vi "main_remote.vi"() -> ()   [LabVIEW 2019]
uses:
  Ctrl/status.ctl
  Ctrl/cmd_common.ctl
  Ctrl/udp_item.ctl
panel:
  out "Lat Long":cluster{"Lat":dbl, "Long":dbl} {"Lat" format="%.8f"; "Long" format="%.8f"}
  out "Batt":dbl(slide) scale=25.0..29.0
  out "Velocity feedback":cluster{"VL-p":dbl, "VA-p":dbl} {"VL-p" scale=-1.0..1.0; "VA-p" scale=-1.0..1.0}
  out "Error Display":T2={"AGV"=2, "AGV Estop"=0, "Obstacle"=2, "GNSS"=1, "TIM571"=1, "Cam"=2, "Joystick"=0}
  out "Connection":i32(ring)=1
  in  "close":bool
  in  "Start":bool
  in  "Stop":bool
  in  "tap UI":enum32{"Main", "Config"}(tab)
  out "Joystick":cluster{"X":dbl, "Y":dbl}[](graph)=[{"X"=0.0, "Y"=0.0}, {"X"=-0.0007812738425855281, "Y"=-0.008435316019165624}]
  in  "agv control":T3
  out "Image 3":T4(plugin-control)
  in  "Joystick cfg":T5={"X axis max"=0.0, "X axis min"=0.0, "Y axis max"=0.0, "Y axis min"=0.0, "Speed-out_max"=0.0, "Speed-out_min"=0.0, "Steer-out_max"=0.0, "Steer-out_min"=0.0, "Joystick ID"=0, "joystick scale"=327670}
  in  "udp cfg":T6={"local port"=61556, "remote port"=61550, "RBA IP"="192.168.1.34"}
  out "udp r buff out":string
  in  "RBA status":string
  out "speed_feedback":cluster{"X":dbl, "Y":dbl}[](graph)=[{"X"=0.0, "Y"=0.0}, {"X"=-0.0007812738425855281, "Y"=-0.008435316019165624}]
  # "SRC Remote"
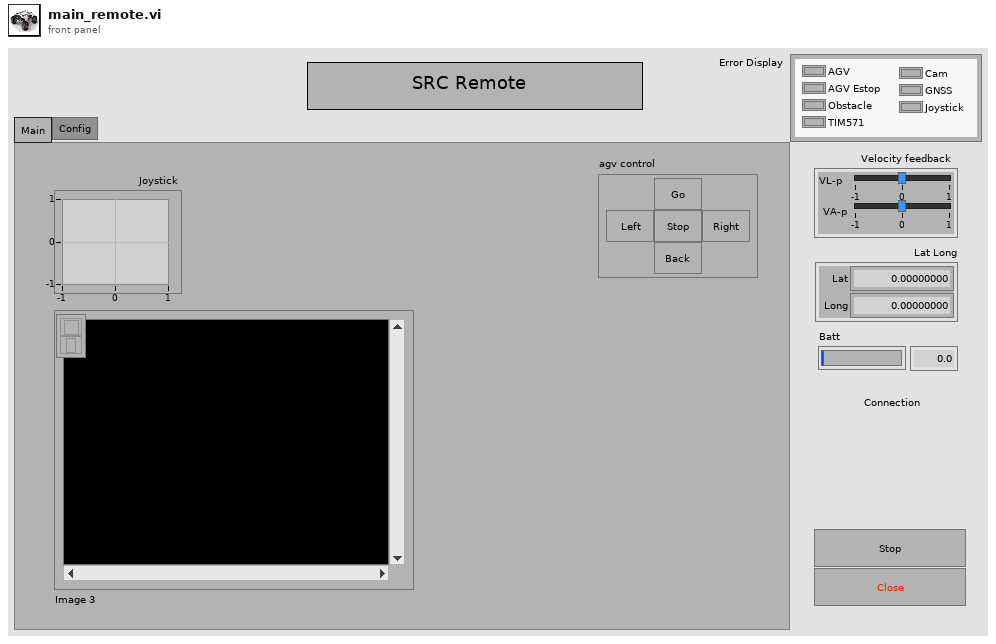
[diagram p1: front panel]
types:
  T1 = typedef "status.ctl" = u16
  T2 = cluster{"AGV":T1, "AGV Estop":T1, "Obstacle":T1, "GNSS":T1, "TIM571":T1, "Cam":T1, "Joystick":T1}
  T3 = cluster{"VL_add":bool, "VL_sub":bool, "Stop":bool, "VL_add 2":bool, "VL_add 3":bool}
  T4 = typedef "IMAQ Image.ctl" = refnum<image>
  T5 = cluster{"X axis max":dbl, "X axis min":dbl, "Y axis max":dbl, "Y axis min":dbl, "Speed-out_max":dbl, "Speed-out_min":dbl, "Steer-out_max":dbl, "Steer-out_min":dbl, "Joystick ID":i32, "joystick scale":i32}
  T6 = cluster{"local port":u16, "remote port":u16, "RBA IP":string}
  T7 = typedef "cmd_common.ctl" = enum16{"read", "write"}
  T8 = typedef "udp_item.ctl" = enum16{"Long", "Lat", "watchdog", "Scoutmini", "RBAstatus", "Err", "ip", "VLp", "VAp", "Batt"}
  T9 = enum16{"enable", "init", "read", "write joystick", "write manual"}
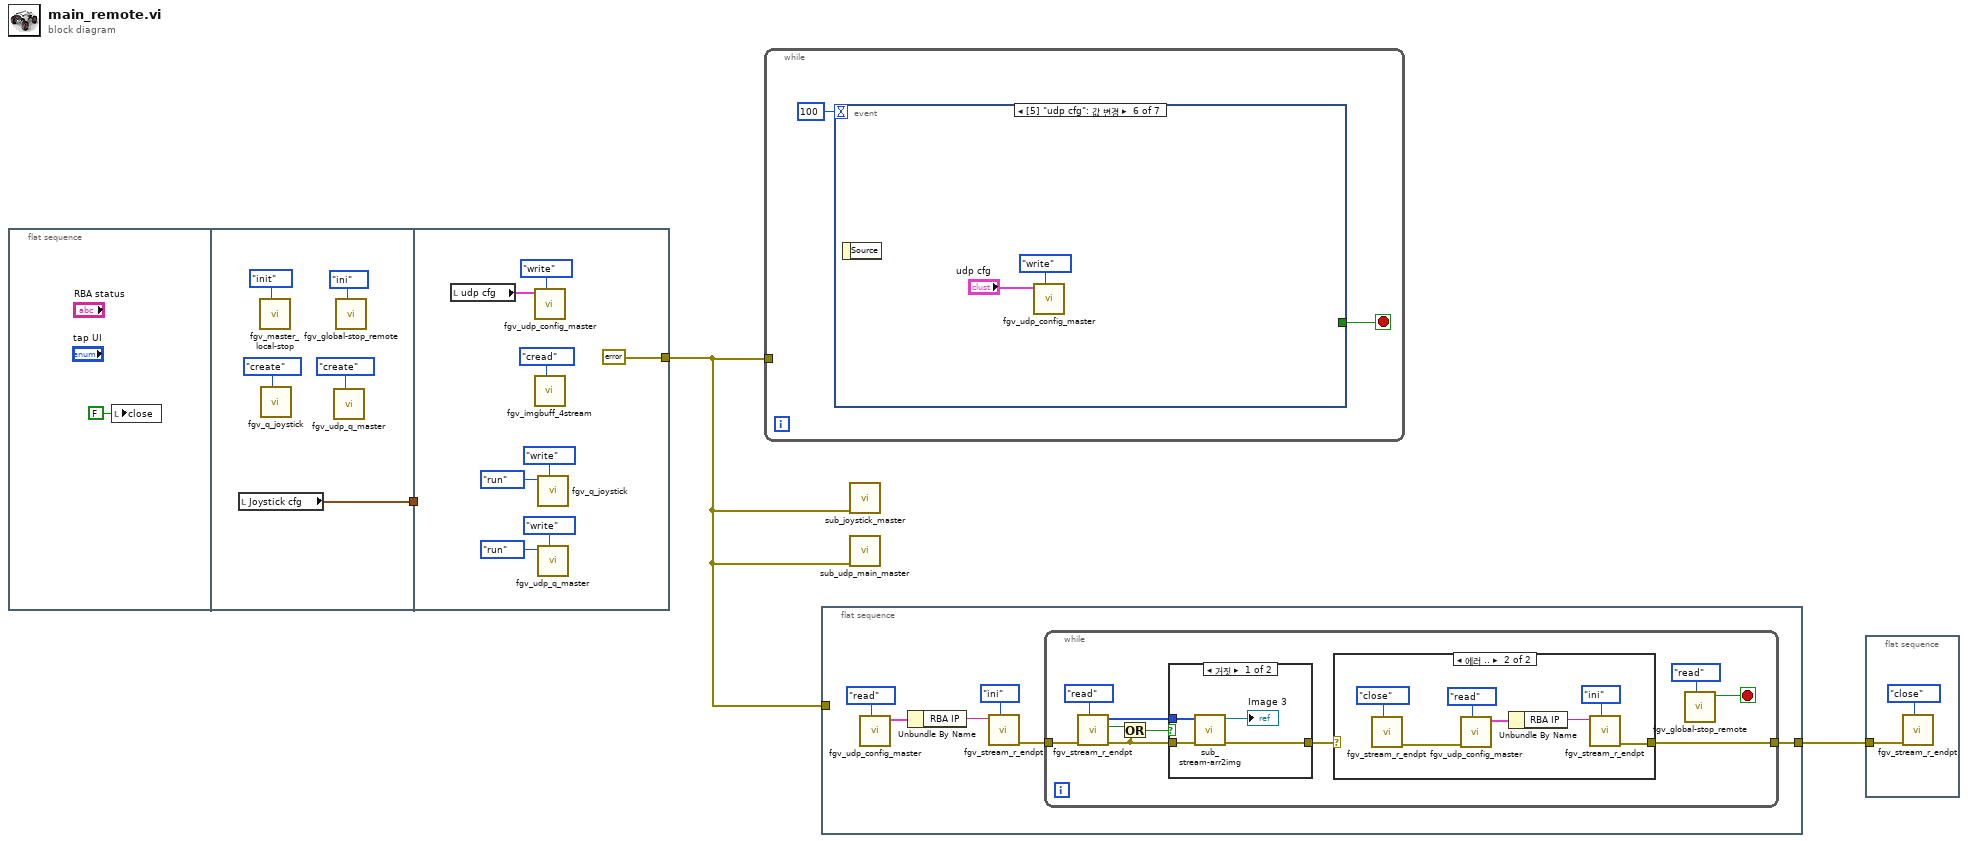
[diagram p0: block diagram]
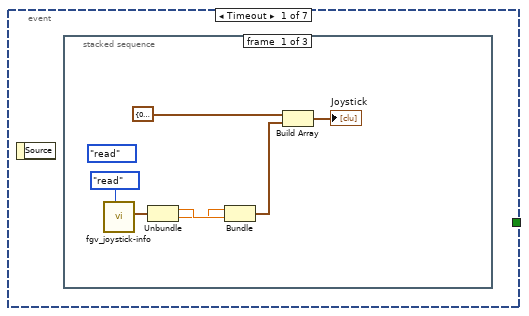
[diagram p4: hidden frame]
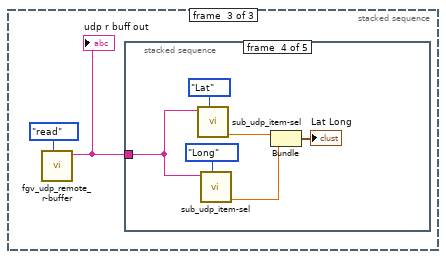
[diagram p6: hidden frame]
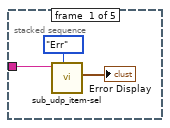
[diagram p7: hidden frame]
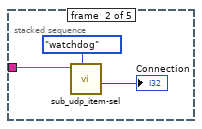
[diagram p8: hidden frame]
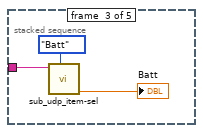
[diagram p9: hidden frame]
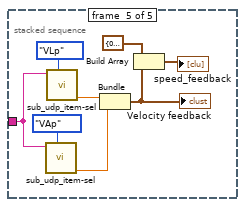
[diagram p10: hidden frame]
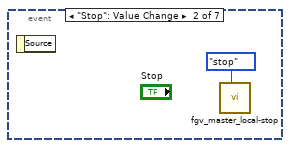
[diagram p11: hidden frame]
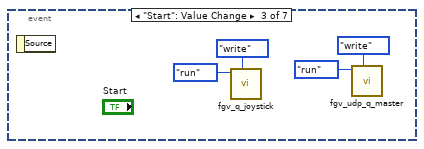
[diagram p12: hidden frame]
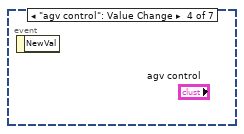
[diagram p13: hidden frame]
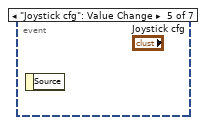
[diagram p14: hidden frame]
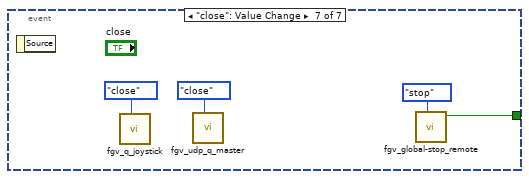
[diagram p15: hidden frame]
diagram:
  n1 = flat-sequence {
    tunnel: [w5] -> w1
    tunnel: [errorcluster {"status"=FALSE, "code"=0, "source"=""} ("error out")] -> w3
    tunnel: w1 -> [_]
    frame #0 {
      n2 = local write "close"(FALSE ("Stop")) -> ()
    }
    frame #1 {
      n3 = local read "Joystick cfg"() -> (w5:T5)
      n4 = call "fgv_master_local-stop.vi"("cmd"=enum16{"init", "read", "stop"}."init") -> ()  [unwired: 10 in, 1 out]
      n5 = call "fgv_q_joystick.vi"("cmd"=enum16{"create", "write", "read", "close"}."create") -> ()  [unwired: 9 in, 2 out]
      n6 = call "fgv_udp_q_master.vi"("cmd"=enum16{"create", "write", "read", "close"}."create") -> ()  [unwired: 9 in, 2 out]
      n7 = call "fgv_global-stop_remote.vi"("cmd"=enum16{"ini", "read", "stop"}."ini") -> ()  [unwired: 10 in, 1 out]
    }
    frame #2 {
      n8 = local read "udp cfg"() -> (w15:T6)
      n9 = call "fgv_udp_config_master.vi"("cmd"=enum16{"write", "read"}."write", "udp cfg"=w15) -> ()  [unwired: 8 in, 2 out]
      n10 = call "fgv_imgbuff_4stream.vi"("cmd"=enum16{"cread", "read", "close"}."cread") -> ()  [unwired: 9 in, 2 out]
      n11 = call "fgv_q_joystick.vi"("cmd"=enum16{"create", "write", "read", "close"}."write", "data"=enum16{"run", "check", "stop"}."run") -> ()  [unwired: 8 in, 2 out]
      n12 = call "fgv_udp_q_master.vi"("cmd"=enum16{"create", "write", "read", "close"}."write", "data"=enum16{"run", "check", "stop"}."run") -> ()  [unwired: 8 in, 2 out]
    }
  }
  n13 = while {
    tunnel: w3 -> [_]
    stop <- w19 stop-if-true
    n14 = event shown="[5] \"udp cfg\": 값 변경" {
      selector: _ -> [_ _ _ _ _ _ _]
      dyn-events: _ -> [_ _ _ _ _ _ _]
      timeout: 100 -> [_ _ _ _ _ _ _]
      tunnel: [_ _ _ _ _ _ w59] -> w19
      event Timeout {
        n15 = event-data() -> ()  [unwired: 1 in, 1 out]
        n16 = stacked-sequence {
          frame #0 {
            (unwired) T9."read" ("init")
            n17 = call "fgv_joystick-info.vi"("init"=enum16{"enable", "init", "read", "write"}."read") -> ("v_val"=w24:cluster{dbl, dbl})  [unwired: 7 in, 3 out]
            n18 = Unbundle(w24) -> (w23:dbl, w22:dbl)
            n19 = Bundle(w22, w23) -> (w21:cluster{dbl, dbl})  [unwired: 1 in]
            n20 = Build Array(cluster{dbl, dbl} {0.0, 0.0} ("원소"), w21) -> (→"Joystick":cluster{dbl, dbl}[])
          }
          frame #1 {
          }
          frame #2 {
            n21 = call "fgv_udp_remote_r-buffer.vi"("cmd"=cmd_common."read") -> ("udp r buff out"=w27:string)  [unwired: 10 in]
            "udp r buff out" <- w27
            n22 = stacked-sequence {
              tunnel: w27 -> [w29 w32 w35 w39 w44]
              frame #0 {
                n23 = call "sub_udp_item-sel.vi"("item"=udp_item."Err", "get-data"=w29) -> ("Error Display"=→"Error Display":T2)  [unwired: 6 in, 3 out]
              }
              frame #1 {
                n24 = call "sub_udp_item-sel.vi"("item"=udp_item."watchdog", "get-data"=w32) -> ("watchdogval"=→"Connection":i32)  [unwired: 6 in, 3 out]
              }
              frame #2 {
                n25 = call "sub_udp_item-sel.vi"("item"=udp_item."Batt", "get-data"=w35) -> ("dbl"=→"Batt":dbl)  [unwired: 6 in, 3 out]
              }
              frame #3 {
                n26 = call "sub_udp_item-sel.vi"("item"=udp_item."Lat", "get-data"=w39) -> ("dbl"=w42:dbl)  [unwired: 6 in, 3 out]
                n27 = call "sub_udp_item-sel.vi"("item"=udp_item."Long", "get-data"=w39) -> ("dbl"=w40:dbl)  [unwired: 6 in, 3 out]
                n28 = Bundle("dbl"=w42, "dbl"=w40) -> (→"Lat Long":cluster{"dbl":dbl, "dbl":dbl})  [unwired: 1 in]
              }
              frame #4 {
                n29 = call "sub_udp_item-sel.vi"("item"=udp_item."VAp", "get-data"=w44) -> ("dbl"=w48:dbl)  [unwired: 6 in, 3 out]
                n30 = call "sub_udp_item-sel.vi"("item"=udp_item."VLp", "get-data"=w44) -> ("dbl"=w49:dbl)  [unwired: 6 in, 3 out]
                n31 = Bundle("dbl"=w49, "dbl"=w48) -> (w51:cluster{"dbl":dbl, "dbl":dbl})  [unwired: 1 in]
                "Velocity feedback" <- w51
                n32 = Build Array(cluster{dbl, dbl} {0.0, 0.0} ("원소"), w51) -> (→"speed_feedback":cluster{"dbl":dbl, "dbl":dbl}[])
              }
            }
          }
        }
      }
      event "Stop": Value Change {
        n33 = event-data() -> ()  [unwired: 1 in, 1 out]
        n34 = call "fgv_master_local-stop.vi"("cmd"=enum16{"init", "read", "stop"}."stop") -> ()  [unwired: 10 in, 1 out]
      }
      event "Start": Value Change {
        n35 = event-data() -> ()  [unwired: 1 in, 1 out]
        n36 = call "fgv_q_joystick.vi"("cmd"=enum16{"create", "write", "read", "close"}."write", "data"=enum16{"run", "check", "stop"}."run") -> ()  [unwired: 8 in, 2 out]
        n37 = call "fgv_udp_q_master.vi"("cmd"=enum16{"create", "write", "read", "close"}."write", "data"=enum16{"run", "check", "stop"}."run") -> ()  [unwired: 8 in, 2 out]
      }
      event "agv control": Value Change {
        n38 = event-data() -> ()  [unwired: 1 in, 1 out]
      }
      event "Joystick cfg": Value Change {
        n39 = event-data() -> ()  [unwired: 1 in, 1 out]
      }
      event "udp cfg": Value Change {
        n40 = event-data() -> ()  [unwired: 1 in, 1 out]
        n41 = call "fgv_udp_config_master.vi"("cmd"=enum16{"write", "read"}."write", "udp cfg"="udp cfg") -> ()  [unwired: 8 in, 2 out]
      }
      event "close": Value Change {
        n42 = event-data() -> ()  [unwired: 1 in, 1 out]
        n43 = call "fgv_q_joystick.vi"("cmd"=enum16{"create", "write", "read", "close"}."close") -> ()  [unwired: 9 in, 2 out]
        n44 = call "fgv_udp_q_master.vi"("cmd"=enum16{"create", "write", "read", "close"}."close") -> ()  [unwired: 9 in, 2 out]
        n45 = call "fgv_global-stop_remote.vi"("cmd"=enum16{"ini", "read", "stop"}."stop") -> ("stop status"=w59:bool)  [unwired: 10 in]
      }
    }
  }
  n46 = flat-sequence {
    tunnel: w3 -> [_]
    tunnel: [w65] -> w2
    frame #0 {
      n47 = call "fgv_udp_config_master.vi"("cmd"=enum16{"write", "read"}."read") -> ("udp cfg out"=w63:T6)  [unwired: 9 in, 1 out]
      n48 = Unbundle By Name(w63) -> ("RBA IP"=w67:string)
      n49 = call "fgv_stream_r_endpt.vi"("cmd"=enum16{"ini", "read", "close"}."ini", "IP Address"=w67) -> ("error out"=w66:errorcluster)  [unwired: 7 in, 2 out]
      n50 = while {
        tunnel: w66 -> [w77]
        tunnel: [w69] -> w65
        stop <- w71 stop-if-true
        n51 = call "fgv_stream_r_endpt.vi"("cmd"=enum16{"ini", "read", "close"}."read", "error in"=w77) -> ("error out"=w73:errorcluster, "time out"=w76:bool, "data_rgb-u8"=w74:u8[])  [unwired: 7 in]
        n52 = Or(x=w76, y=w73) -> (x .or. y?=w75:bool)
        n53 = case shown="거짓" w75 {
          tunnel: w74 -> [w90 _]
          tunnel: [w88 w91] -> w70
          tunnel: w73 -> [w87 w91]
          frame False {
            n54 = call "sub_stream-arr2img.vi"("error in"=w87, "imgarr"=w90) -> ("error out"=w88:errorcluster, "Image Dst Out"=→"Image 3":T4)  [unwired: 8 in]
          }
          frame True {
          }
        }
        n55 = case shown="에러 .." w70 {
          selector: w70 -> [w79 _]
          tunnel: [w79 w80] -> w69
          frame No Error {
          }
          frame Error {
            n56 = call "fgv_stream_r_endpt.vi"("cmd"=enum16{"ini", "read", "close"}."close") -> ("error out"=w81:errorcluster)  [unwired: 8 in, 2 out]
            n57 = call "fgv_udp_config_master.vi"("cmd"=enum16{"write", "read"}."read", "error in"=w81) -> ("udp cfg out"=w86:T6)  [unwired: 8 in, 1 out]
            n58 = Unbundle By Name(w86) -> ("RBA IP"=w84:string)
            n59 = call "fgv_stream_r_endpt.vi"("cmd"=enum16{"ini", "read", "close"}."ini", "IP Address"=w84) -> ("error out"=w80:errorcluster)  [unwired: 7 in, 2 out]
          }
        }
        n60 = call "fgv_global-stop_remote.vi"("cmd"=enum16{"ini", "read", "stop"}."read") -> ("stop status"=w71:bool)  [unwired: 10 in]
      }
    }
  }
  n61 = call "sub_joystick_master.vi"("error in"=w3) -> ()  [unwired: 10 in, 1 out]
  n62 = call "sub_udp_main_master.vi"("error in"=w3) -> ()  [unwired: 10 in, 1 out]
  n63 = flat-sequence {
    tunnel: w2 -> [w92]
    frame #0 {
      n64 = call "fgv_stream_r_endpt.vi"("cmd"=enum16{"ini", "read", "close"}."close", "error in"=w92) -> ()  [unwired: 7 in, 3 out]
    }
  }
